vi "setNodeAttribute.vi"(8 "error in (no error)":errorcluster, 9 "open nodes":refnum<class "xmlNode.lvclass">[](array[class]), 10 "open names":string[](array[string]), 11 "name in":string) -> (0 "error out":errorcluster, 1 "open nodes out":refnum<class "xmlNode.lvclass">[](array[class]), 2 "open names out":string[](array[string]), 3 "name out":string)   [LabVIEW 2009, in "Tools.lvlib" / "xml.lvlib" / "XmlParser.lvclass"]
uses:
  XmlParser.lvclass
  xmlNode/xmlNode.lvclass
panel:
  out "Numeric":i32
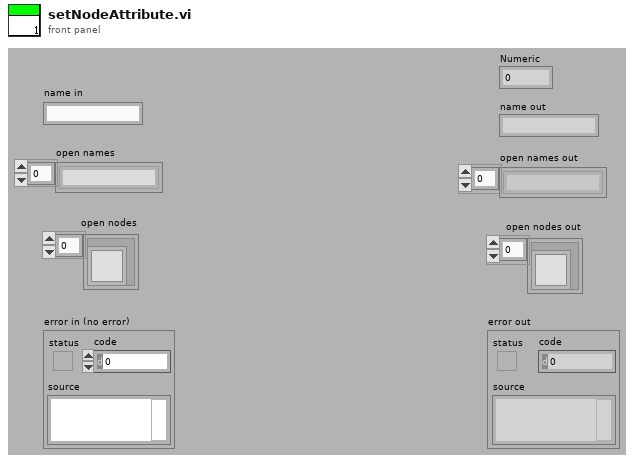
[diagram p1: front panel]
types:
  T1 = cluster{"result string":string, "result string":string}
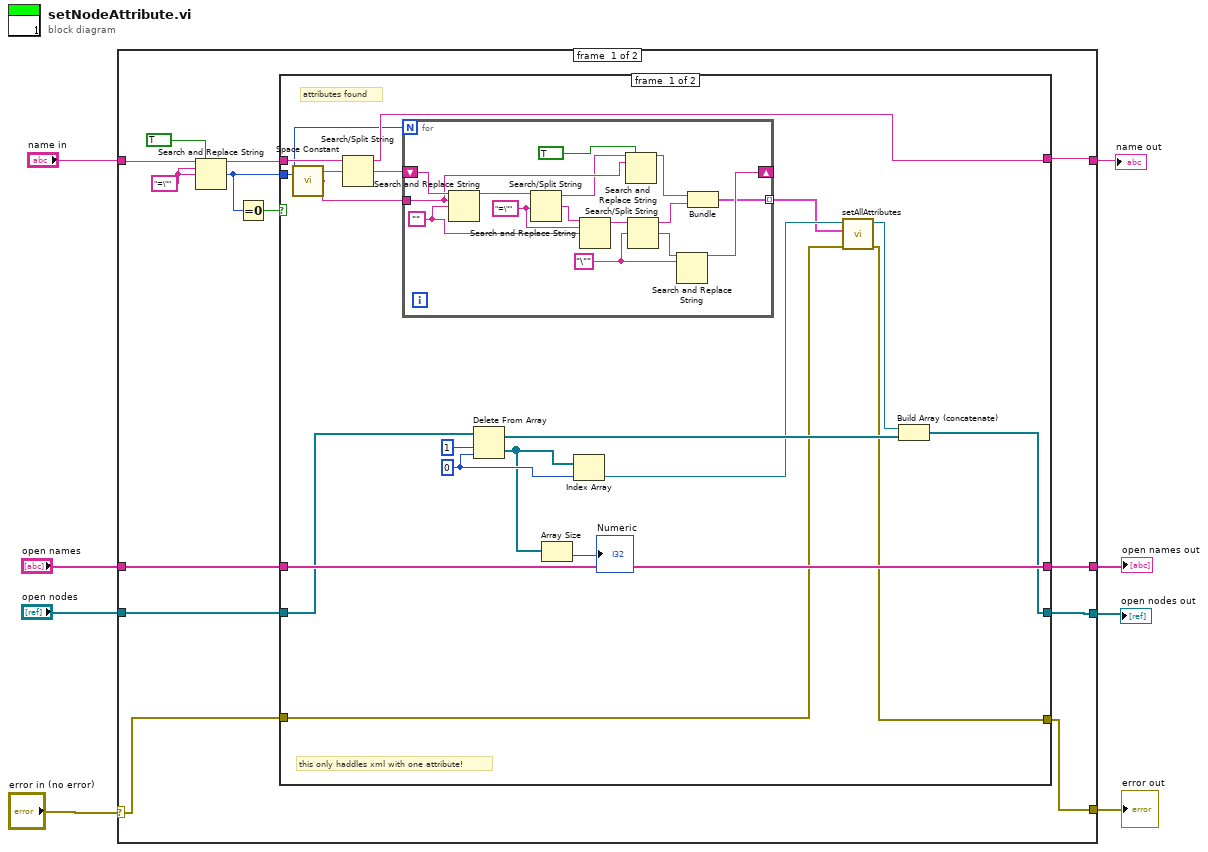
[diagram p0: block diagram]
diagram:
  n1 = case shown="No Error" "error in (no error)" {
    selector: "error in (no error)" -> [w12 w62]
    tunnel: [w11 w62] -> w7
    tunnel: "name in" -> [w21 w61]
    tunnel: "open names" -> [w16 w60]
    tunnel: "open nodes" -> [w15 w59]
    tunnel: [w17 w61] -> w1
    tunnel: [w14 w60] -> w3
    tunnel: [w13 w59] -> w2
    frame #0 {
      w20 = "=\""
      n2 = Search and Replace String(replace all?=TRUE, input string=w21, search string=w20, replace string=w20) -> (result string=w18:string, number of replacements=w10:i32)  [unwired: 4 in, 2 out]
      n3 = Equal To 0?(x=w10) -> (x = 0?=w19:bool)
      n4 = case shown="False" w19 {
        tunnel: w18 -> [w39 w58]
        tunnel: [w38 w58] -> w17
        tunnel: w16 -> [w37 w57]
        tunnel: w15 -> [w36 w56]
        tunnel: [w37 w57] -> w14
        tunnel: [w34 w56] -> w13
        tunnel: w12 -> [w25 w55]
        tunnel: [w24 w55] -> w11
        tunnel: w10 -> [w22 _]
        frame #0 {
          w33 = 0
          # "attributes found"
          # "this only haddles xml with one attribute!"
          n5 = call <vilib>:"Space Constant.vi"() -> ("String"=w28:string)
          n6 = Search/Split String(string=w39, search string/char (-)=w28) -> (substring before match=w38:string, match + rest of string=w29:string)  [unwired: 1 in, 1 out]
          n7 = for {
            N: w22 -> [_]
            tunnel: w28 -> [w43]
            shift-right: [w45] -> _
            shift-left: w29 -> [w54]
            tunnel: [w44] -> w23 mode=indexing
            w48 = "\""
            w51 = "=\""
            w50 = ""
            n8 = Search and Replace String(input string=w54, search string=w43, replace string=w50) -> (result string=w53:string)  [unwired: 5 in, 3 out]
            n9 = Search/Split String(string=w53, search string/char (-)=w51) -> (substring before match=w41:string, match + rest of string=w52:string)  [unwired: 1 in, 1 out]
            n10 = Search and Replace String(input string=w52, search string=w51, replace string=w50) -> (result string=w49:string)  [unwired: 5 in, 3 out]
            n11 = Search and Replace String(replace all?=TRUE, input string=w41, search string=w43) -> (result string=w40:string)  [unwired: 5 in, 3 out]
            n12 = Search/Split String(string=w49, search string/char (-)=w48) -> (substring before match=w47:string, match + rest of string=w46:string)  [unwired: 1 in, 1 out]
            n13 = Search and Replace String(input string=w46, search string=w48) -> (result string=w45:string)  [unwired: 6 in, 3 out]
            n14 = Bundle("result string"=w40, "result string"=w47) -> (w44:T1)  [unwired: 1 in]
          }
          n15 = Delete From Array(array=w36, length=1, index=w33) -> (deleted portion=w32:refnum<class "xmlNode.lvclass">[], array with subset deleted=w30:refnum<class "xmlNode.lvclass">[])
          n16 = Array Size(array=w32) -> (size(s)=→"Numeric":i32)
          n17 = Index Array(array=w32, index=w33) -> (element=w27:refnum<class "xmlNode.lvclass">)
          n18 = call-dynamic "setAllAttributes.vi"("error in (no error)"=w25, "attributes"=w23, "xmlNode in"=w27) -> ("error out"=w24:errorcluster, "xmlNode out"=w26:refnum<class "xmlNode.lvclass">)  [unwired: 7 in]
          n19 = Build Array (concatenate)(w26, w30) -> (w34:refnum<class "xmlNode.lvclass">[])
        }
        frame #1 {
          # "no attributes found"
        }
      }
    }
    frame #1 {
    }
  }
  "error out" <- w7
  "open nodes out" <- w2
  "open names out" <- w3
  "name out" <- w1
